vi "Example Analog 1.vi"(8 "Error In":errorcluster) -> (0 "Error Out":errorcluster)   [LabVIEW 2018]
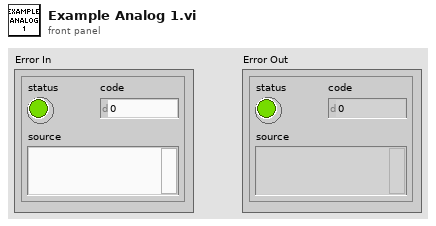
[diagram p1: front panel]
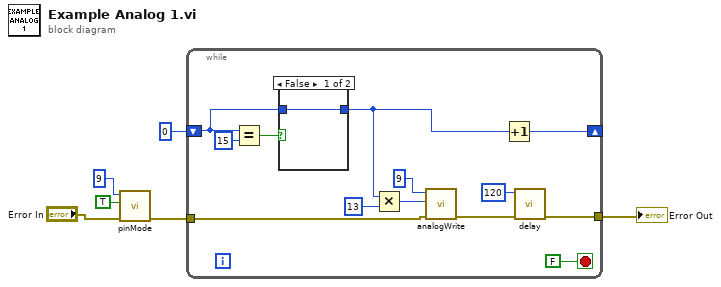
[diagram p0: block diagram]
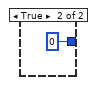
[diagram p2: hidden frame]
diagram:
  n1 = call "pinMode.vi"("Error In"="Error In", "output?"=TRUE, "pin number"=9) -> ("Error Out"=w5:errorcluster)  [unwired: 8 in]
  n2 = while {
    tunnel: w5 -> [w14]
    tunnel: [w16] -> w3
    shift-right: [w13] -> _
    shift-left: 0 ("pin number") -> [w10]
    stop <- FALSE stop-if-true
    n3 = Equal?(x=w10, y=15) -> (x = y?=w12:bool)
    n4 = case shown="False" w12 {
      tunnel: w10 -> [w20 _]
      tunnel: [w20 0 ("pin number")] -> w8
      frame False {
      }
      frame True {
      }
    }
    n5 = Multiply(x=w8, y=13) -> (x*y=w9:i32)
    n6 = call "analogWrite.vi"("Error In"=w14, "value"=w9, "pin number"=9) -> ("Error Out"=w18:errorcluster)  [unwired: 8 in]
    n7 = Increment(x=w8) -> (x+1=w13:i32)
    n8 = call "delay.vi"("Error In"=w18, "time (ms)"=120) -> ("Error Out"=w16:errorcluster)  [unwired: 9 in]
  }
  "Error Out" <- w3
